vi "ECG - Fast Fourier Transform.vi"() -> ()   [LabVIEW 2013]
uses:
  <vilib>/addons/Biomedical/Biosignal Measurements/ECG/HRV analysis/subVIs/bmt_HRV FFT Settings.ctl
  <vilib>/addons/Biomedical/Biosignal Measurements/ECG/HRV analysis/subVIs/bmt_HRV Frequency Bands.ctl
  <vilib>/addons/Biomedical/Controls/Biosignal/Biosignal Spectrum/Biosignal Spectrum.xctl
  <vilib>/addons/Biomedical/Biosignal Measurements/ECG/HRV analysis/HRV FFT Spectrum (Waveform Evenly Sampled RR).vi
  <vilib>/addons/Biomedical/Controls/Biosignal/HRV Spectrum Helper (FFT).vi
  <vilib>/addons/Biomedical/NI_BMTK_Measurements.lvlib
  <vilib>/addons/Biomedical/NI_BMTK_Controls.lvlib
panel:
  out "Signal pre analize":waveform(dbl)[](graph)
  out "Lokacija sacuvanog fajla na racunaru":path
  out "FFT Spektar":cluster{"f0":dbl, "df":dbl, "S(f)":dbl[]}(xcontrol)
  out "VLF Snaga (FFT)":dbl format="%#_2f ms^2"
  out "LF Snaga (FFT)":dbl format="%#_2f ms^2"
  out "HF Snaga (FFT)":dbl format="%#_2f ms^2"
  out "VLF [%] (FFT)":dbl format="%#_2f %"
  out "LF [%] (FFT)":dbl format="%#_2f %"
  out "HF [%] (FFT)":dbl format="%#_2f %"
  out "LF norm (FFT)":dbl format="%#_3f n.u."
  out "HF norm (FFT)":dbl format="%#_3f n.u."
  out "LF/HF (FFT)":dbl format="%#_2f"
  in  "FFT podesavanja":T1={"podesavanja prozora"={"vrsta prozora"=1, "duzina"=1024, "preklapanje [%]"=50.0}, "frekventni opsezi"={"VLF high"=0.04, "VLF low"=0.0, "LF high"=0.15, "LF low"=0.04, "HF high"=0.4, "HF low"=0.15}, "dB on? (F)"=FALSE, "frekventni binovi"=1024} {"podesavanja prozora"."vrsta prozora" items=["None ", "Hanning", "Hamming", "Blackman-Harris", "Exact Blackman", "Blackman", "Flat Top", "4 Term B-Harris ", "7 Term B-Harris", "Low Sidelobe"]}
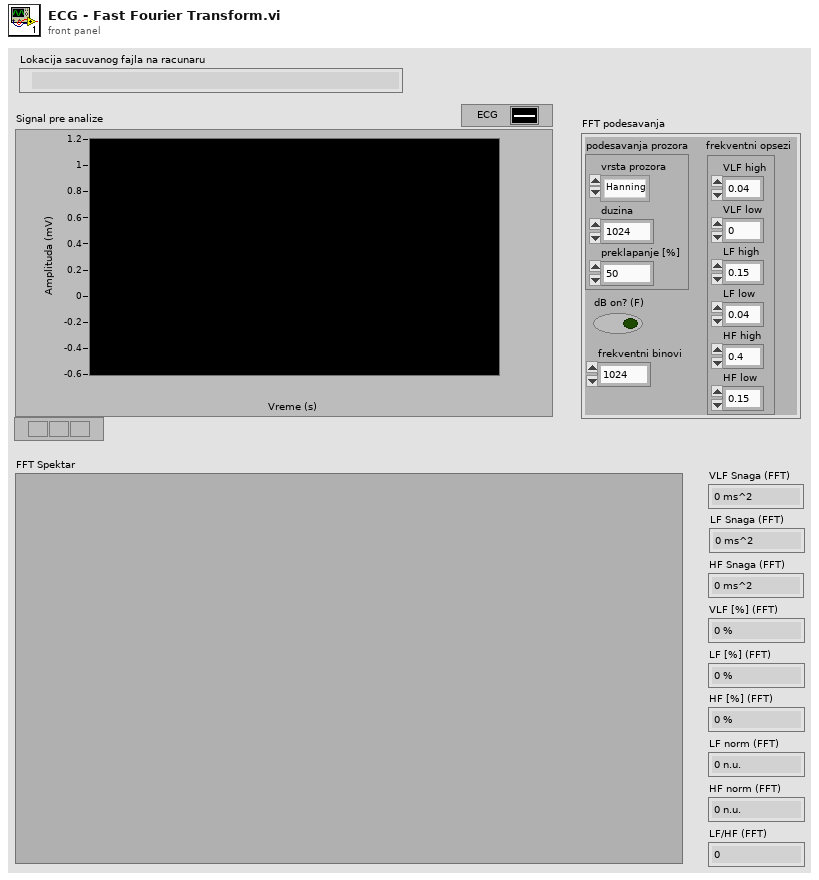
[diagram p1: front panel]
types:
  T1 = typedef "NI_BMTK_Measurements.lvlib/bmt_HRV FFT Settings.ctl" = cluster{"podesavanja prozora":cluster{"vrsta prozora":u16, "duzina":i32, "preklapanje [%]":dbl}, "frekventni opsezi":T2, "dB on? (F)":bool, "frekventni binovi":i32}
  T2 = typedef "NI_BMTK_Measurements.lvlib/bmt_HRV Frequency Bands.ctl" = cluster{"VLF high":dbl, "VLF low":dbl, "LF high":dbl, "LF low":dbl, "HF high":dbl, "HF low":dbl}
  T3 = enum16{"open", "open or create", "create or replace", "create", "open (read-only)"}
  T4 = typedef "NI_BMTK_Measurements.lvlib/bmt_Spectrum Meatures.ctl" = cluster{"VLF peak frequency":dbl, "VLF peak amplitude ":dbl, "LF peak frequency ":dbl, "LF peak amplitude ":dbl, "HF peak frequency":dbl, "HF peak amplitude":dbl, "VLF power":dbl, "LF power":dbl, "HF power":dbl, "LF norm":dbl, "HF norm":dbl, "LF/HF":dbl, "VLF [%]":dbl, "LF [%]":dbl, "HF [%]":dbl}
  T5 = enum16{"open", "replace", "create", "open or create", "replace or create", "replace or create with confirmation"}
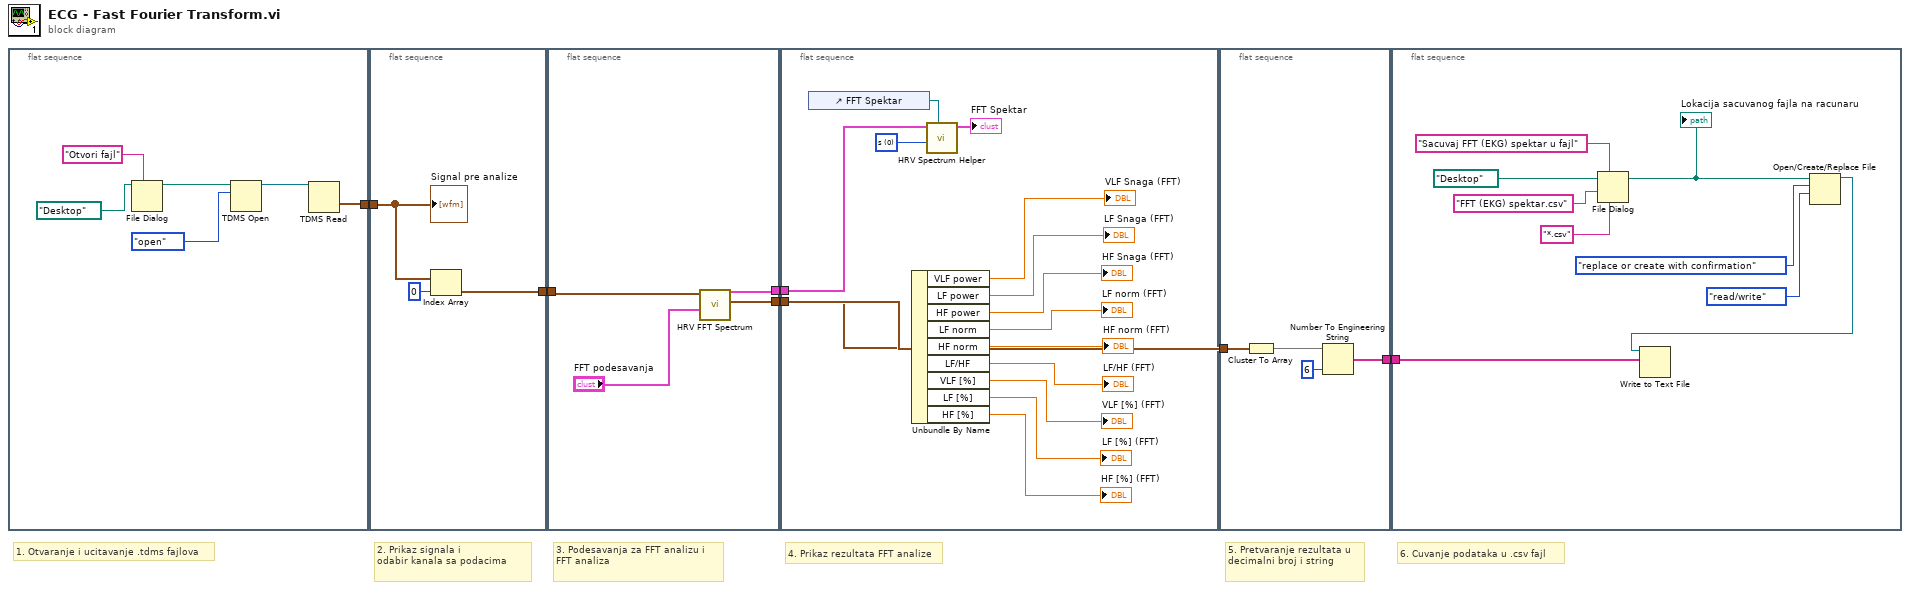
[diagram p0: block diagram]
diagram:
  # "6. Cuvanje podataka u .csv fajl"
  # "5. Pretvaranje rezultata u decimalni broj i string"
  # "4. Prikaz rezultata FFT analize"
  # "3. Podesavanja za FFT analizu i FFT analiza"
  # "2. Prikaz signala i \nodabir kanala sa podacima"
  # "1. Otvaranje i ucitavanje .tdms fajlova"
  n1 = flat-sequence {
    tunnel: [w7] -> w2
    frame #0 {
      n2 = File Dialog(7:"Otvori fajl" ("prompt"), 11:path "/Desktop" ("start path")) -> (3:w9:path)  [unwired: 2 in, 6 out]
      n3 = TDMS Open(10:T3."open" ("operation (0:open)"), 11:w9) -> (3:w10:refnum<k34>)  [unwired: 5 in, 1 out]
      n4 = TDMS Read(0:w10) -> (10:w7:waveform(dbl)[])  [unwired: 7 in, 5 out]
    }
  }
  n5 = flat-sequence {
    tunnel: w2 -> [w14]
    tunnel: [w12] -> w1
    frame #0 {
      n6 = Index Array(array=w14, index=0) -> (element=w12:waveform(dbl))
      "Signal pre analize" <- w14
    }
  }
  n7 = flat-sequence {
    tunnel: [w18] -> w5
    tunnel: [w16] -> w4
    tunnel: w1 -> [w15]
    frame #0 {
      n8 = call-poly <vilib>:"HRV FFT Spectrum.vi"("FFT settings"="FFT podesavanja", "RR"=w15) -> ("FFT measurements"=w16:T4, "FFT spectrum"=w18:cluster{"f0":dbl, "df":dbl, "S(f)":dbl[]})  [unwired: 7 in, 1 out]
    }
  }
  n9 = flat-sequence {
    tunnel: w5 -> [w29]
    tunnel: w4 -> [w20]
    frame #0 {
      w30 = u16 0 items=["s", "ms"] ("RR unit")
      n10 = control-ref of="FFT Spektar"() -> (w31:refnum<vi>)
      n11 = Unbundle By Name(w20) -> ("VLF power"=→"VLF Snaga (FFT)":dbl, "LF power"=→"LF Snaga (FFT)":dbl, "HF power"=→"HF Snaga (FFT)":dbl, "LF norm"=→"LF norm (FFT)":dbl, "HF norm"=→"HF norm (FFT)":dbl, "LF/HF"=→"LF/HF (FFT)":dbl, "VLF [%]"=→"VLF [%] (FFT)":dbl, "LF [%]"=→"LF [%] (FFT)":dbl, "HF [%]"=→"HF [%] (FFT)":dbl)
      n12 = call-poly <vilib>:"HRV Spectrum Helper.vi"("HRV spectrum"=w31, "RR unit"=w30, "spectrum in"=w29) -> ("spectrum out"=→"FFT Spektar":cluster{"f0":dbl, "df":dbl, "S(f)":dbl[]})  [unwired: 7 in, 1 out]
    }
  }
  n13 = flat-sequence {
    tunnel: w4 -> [w36]
    tunnel: [w35] -> w3
    frame #0 {
      n14 = Cluster To Array(cluster=w36) -> (array=w34:dbl[])
      n15 = Number To Engineering String(2:i16 6 ("precision (6)"), 4:w34) -> (0:w35:string[])  [unwired: 2 in]
    }
  }
  n16 = flat-sequence {
    tunnel: w3 -> [w37]
    frame #0 {
      n17 = File Dialog(6:"*.csv" ("pattern (all files)"), 7:"Sacuvaj FFT (EKG) spektar u fajl" ("prompt"), 9:"FFT (EKG) spektar.csv" ("default name"), 11:path "/Desktop" ("start path")) -> (3:w40:path)  [unwired: 1 in, 5 out]
      "Lokacija sacuvanog fajla na racunaru" <- w40
      n18 = Open/Create/Replace File(file path (use dialog)=w40, operation (0:open)=T5."replace or create with confirmation", access (0:read/write)=enum16{"read/write", "read-only", "write-only"}."read/write") -> (refnum out=w38:refnum<file>)  [unwired: 3 in, 2 out]
      n19 = Write to Text File(file (use dialog)=w38, text=w37) -> ()  [unwired: 2 in, 3 out]
    }
  }
